vi "U3 easy Stream Example Full.vi"() -> ()   [LabVIEW 2021]
panel:
  out "Stream Parameters":T1 {"Device Backlog [%]" format="%.2f"}
  in  "PC buffer size (seconds)":dbl=10.0 format="%.2f"
  in  "Scan List (-)":u8[](array[numeric])=[31, 31, 31, 31, 31, 31, 31, 31, 31, 31, 31, 31, 31, 31, 31, 31, 31, 31, 31, 31, 31, 31, 31, 31, 31, 31, 31, 31, 31, 31, 31, 31, 31, 31, 31, 31, 31, 31, 31, 31, 31, 31, 31, 31, 31, 31, 31, 31, 31, 31, 31, 31, 31, 31, 31, 31, 31, 31, 31, 31, 31, 31, 31, 31, 31, 31, 31, 31, 31, 31, 31, 31, 31, 31, 31, 31, 31, 31, 31, 31, 31, 31, 31, 31, 31, 31, 31, 31, 31, 31, 31, 31, 31, 31, 31, 31, 31, 31, 31, 31, 31, 31, 31, 31, 31, 31, 31, 31, 31, 31, 31, 31, 31, 31, 31, 31, 31, 31, 31, 31, 31, 31, 31, 31, 31, 31, 31, 31]
  out "Data":dbl[][](array[numeric]) format="%.3f"
  out "Waveform Graph":dbl[][](graph)
  in  "Scan List (+)":u8[](array[numeric])=[0, 1, 2, 3]
  out "# of iterations":i32
  in  "Scan Rate (Hz)":dbl=1000.0 format="%.3f"
  in  "stop":bool
  out "Error Message":string
  # "This example streams from the first found USB U3.  Streaming\nrequires U3 hardware revision 1.21+."
  # "The + scan list is the positive\nchannels.  For each element in\nthe + list, there must also be\nan element in the - list, which is\nthe negative channels.  For\nsingle-ended channels, put in\n31 for the negative channel.\n\nTo remove an element, right-click\non it, select Data Operations =>\nRemove Element.\n\nTo empty an array, right-click\nnear the edge, select Data\nOperations => Empty Array.\n\nOther useful operations:  From the\nOperate menu are \"Make Current\nValues Default\" and \"Reinitialize\nTo Default\"."
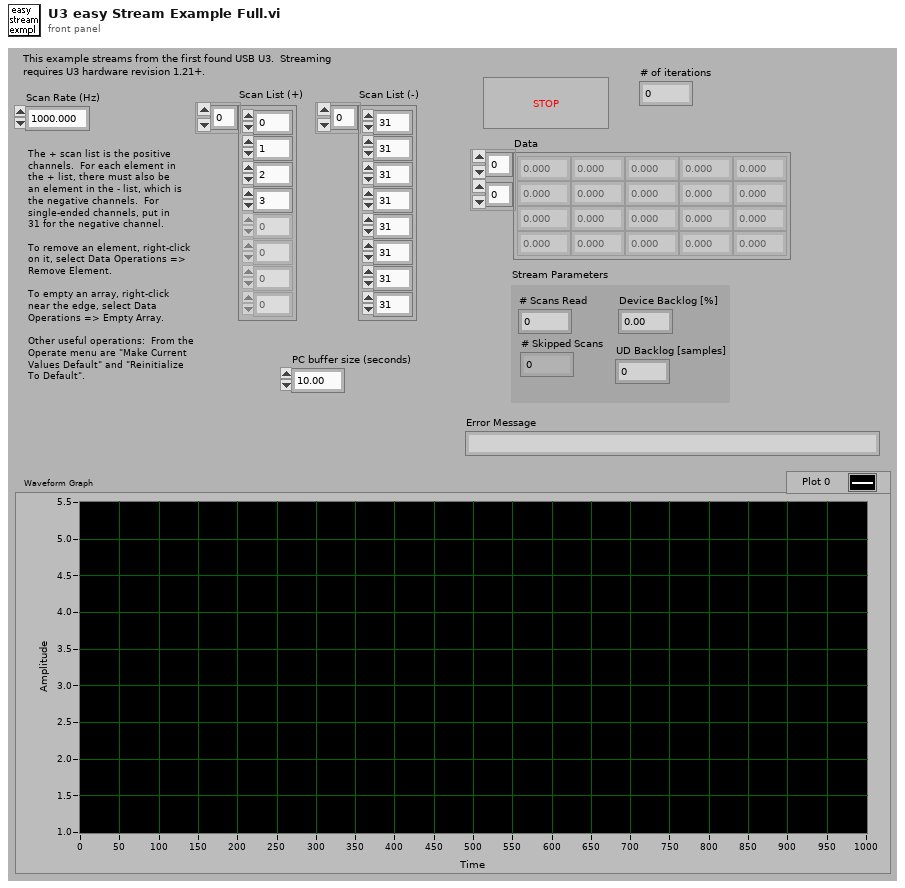
[diagram p1: front panel]
types:
  T1 = cluster{"# Scans Read":i32, "# Skipped Scans":i32, "Device Backlog [%]":dbl, "UD Backlog [samples]":i32}
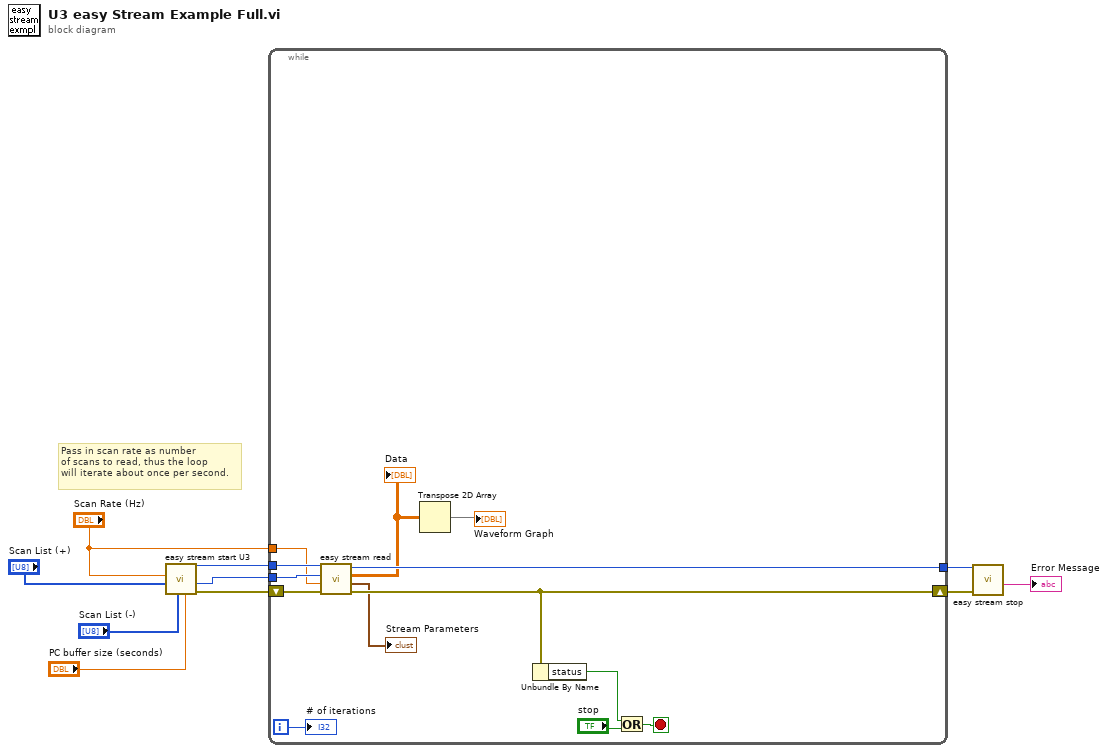
[diagram p0: block diagram]
diagram:
  # "Pass in scan rate as number\nof scans to read, thus the loop\nwill iterate about once per second."
  n1 = call <vilib>:"easy stream start U3.vi"("PC buffer size (seconds)"="PC buffer size (seconds)", "Scan List (-)"="Scan List (-)", "Scan List (+)"="Scan List (+)", "Scan Rate (Hz)"="Scan Rate (Hz)") -> ("error out"=w10:errorcluster, "# Channels"=w8:i32, "Handle Out"=w7:i32)  [unwired: 4 in, 1 out]
  n2 = while {
    tunnel: "Scan Rate (Hz)" -> [w12]
    tunnel: [w15] -> w5
    tunnel: w7 -> [w16]
    tunnel: w8 -> [w17]
    shift-left: w10 -> [w18]
    shift-right: [w13] -> w6
    i -> [w20]
    stop <- w21 stop-if-true
    n3 = call <vilib>:"easy stream read.vi"("error in"=w18, "Scans To Read"=w12, "# Channels In Stream"=w17, "Handle In"=w16) -> ("error out"=w13:errorcluster, "Stream Parameters"=→"Stream Parameters":T1, "Data"=w14:dbl[][], "Handle Out"=w15:i32)  [unwired: 4 in]
    "Data" <- w14
    n4 = Transpose 2D Array(2D array=w14) -> (transposed array=→"Waveform Graph":dbl[][])
    n5 = Unbundle By Name(w13) -> ("status"=w22:bool)
    n6 = Or(x=w22, y="stop") -> (x .or. y?=w21:bool)
    "# of iterations" <- w20
  }
  n7 = call <vilib>:"easy stream stop.vi"("error in"=w6, "Handle In"=w5) -> ("Error Message"=→"Error Message":string)  [unwired: 7 in, 2 out]
